vi "IIR Cascade Filter PtByPt.vi"(2 "initialize":bool, 3 "IIR Filter Cluster":T1, 5 "x":dbl format="%0.2f") -> (0 "error":i32, 1 "Filtered x":dbl format="%0.2f")   [LabVIEW 2020, in "NI_PtbyPt.lvlib"]
doc: "Filters <B>x</B> using the cascade form of the IIR filter specified by the <B>IIR Filter Cluster</B>."
uses:
  NI_PtbyPt.lvlib
  IIR Cascade Filter (DBL).vi
  NI_AALBase.lvlib
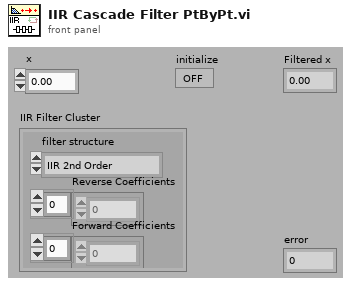
[diagram p1: front panel]
types:
  T1 = cluster{"filter structure":enum32{"IIR 2nd Order", "IIR 4th Order"}, "Reverse Coefficients":dbl[], "Forward Coefficients":dbl[]}
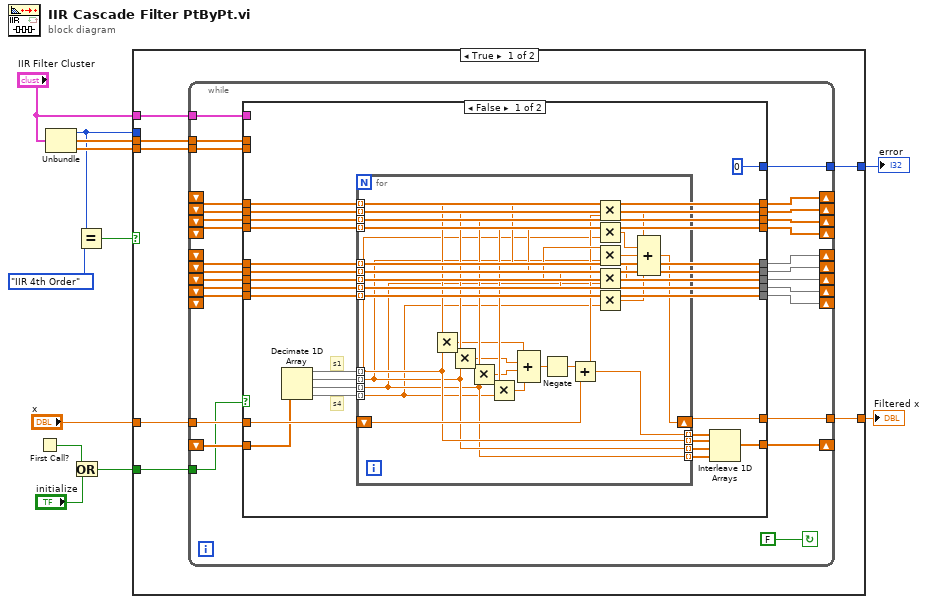
[diagram p0: block diagram]
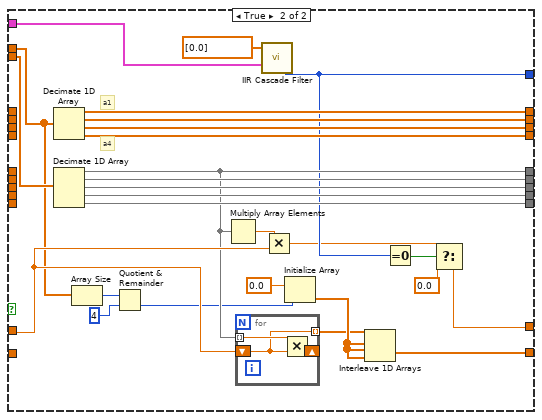
[diagram p2: hidden frame]
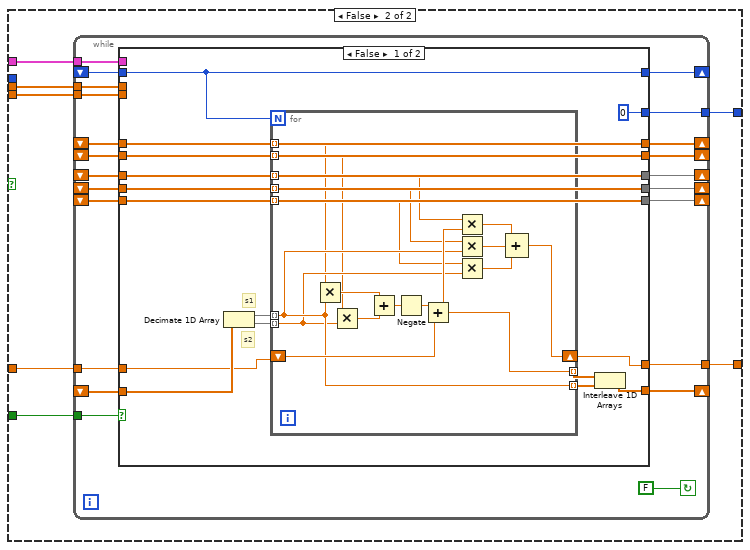
[diagram p3: hidden frame]
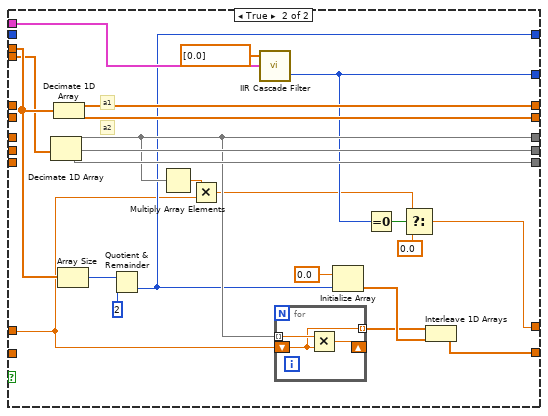
[diagram p4: hidden frame]
diagram:
  n1 = First Call?() -> (First Call?: T/F=w4:bool)
  n2 = Unbundle("IIR Filter Cluster") -> ("filter structure"=w9:enum32{"IIR 2nd Order", "IIR 4th Order"}, "Reverse Coefficients"=w10:dbl[], "Forward Coefficients"=w11:dbl[])
  n3 = Or(x=w4, y="initialize") -> (x .or. y?=w5:bool)
  n4 = Equal?(x=w9, y=enum32{"IIR 2nd Order", "IIR 4th Order"}."IIR 4th Order") -> (x = y?=w7:bool)
  n5 = case shown="True" w7 {
    tunnel: "x" -> [w18 w132]
    tunnel: w11 -> [w16 w130]
    tunnel: w9 -> [_ _]
    tunnel: w10 -> [w17 w131]
    tunnel: [w15 w129] -> w6
    tunnel: w5 -> [w19 w133]
    tunnel: "IIR Filter Cluster" -> [w14 w128]
    tunnel: [w13 w127] -> w2
    frame True {
      n6 = while {
        tunnel: [w21] -> w13
        tunnel: w14 -> [w22]
        tunnel: [w25] -> w15
        shift-left: _ -> [w26]
        shift-right: [w24] -> _
        shift-left: _ -> [w27]
        shift-right: [w28] -> _
        shift-left: _ -> [w29]
        shift-right: [w31] -> _
        shift-left: _ -> [w30]
        shift-right: [w32] -> _
        shift-left: _ -> [w33]
        shift-right: [w34] -> _
        tunnel: w18 -> [w35]
        tunnel: w17 -> [w36]
        shift-left: _ -> [w37]
        shift-right: [w39] -> _
        shift-left: _ -> [w38]
        shift-right: [w40] -> _
        shift-left: _ -> [w42]
        shift-right: [w45] -> _
        shift-left: _ -> [w41]
        shift-right: [w44] -> _
        shift-left: _ -> [w43]
        shift-right: [w46] -> _
        tunnel: w16 -> [w47]
        tunnel: w19 -> [w20]
        stop <- FALSE continue-if-true
        n7 = case shown="False" w20 {
          tunnel: w47 -> [_ w112]
          tunnel: [w64 w119] -> w46
          tunnel: [w63 w118] -> w45
          tunnel: [w62 w117] -> w44
          tunnel: w43 -> [w64 _]
          tunnel: w42 -> [w63 _]
          tunnel: w41 -> [w62 _]
          tunnel: [w67 w121] -> w40
          tunnel: [w66 w120] -> w39
          tunnel: w38 -> [w67 _]
          tunnel: w37 -> [w66 _]
          tunnel: w36 -> [_ w100]
          tunnel: w35 -> [w56 w110]
          tunnel: [w68 w122] -> w34
          tunnel: w33 -> [w68 _]
          tunnel: [w65 w109] -> w32
          tunnel: [w61 w116] -> w31
          tunnel: w30 -> [w65 _]
          tunnel: w29 -> [w61 _]
          tunnel: [w69 w123] -> w28
          tunnel: w27 -> [w69 _]
          tunnel: [w54 w102] -> w25
          tunnel: w26 -> [w55 _]
          tunnel: [w49 w111] -> w24
          tunnel: w22 -> [_ w107]
          tunnel: [0 ("error") w105] -> w21
          frame False {
            # "s4"
            # "s1"
            n8 = Decimate 1D Array(w55) -> (w60:dbl[], w59:dbl[], w58:dbl[], w57:dbl[])
            n9 = for {
              tunnel: w67 -> [w94] mode=indexing
              tunnel: w66 -> [w93] mode=indexing
              tunnel: w64 -> [w85] mode=indexing
              tunnel: w63 -> [w84] mode=indexing
              tunnel: w62 -> [w83] mode=indexing
              tunnel: w68 -> [w95] mode=indexing
              tunnel: w61 -> [w82] mode=indexing
              tunnel: w69 -> [w96] mode=indexing
              tunnel: w65 -> [w86] mode=indexing
              tunnel: w60 -> [w73] mode=indexing
              tunnel: w59 -> [w72] mode=indexing
              tunnel: w58 -> [w71] mode=indexing
              tunnel: w57 -> [w70] mode=indexing
              tunnel: [w74] -> w53 mode=indexing
              tunnel: [w71] -> w50 mode=indexing
              tunnel: [w72] -> w51 mode=indexing
              tunnel: [w73] -> w52 mode=indexing
              shift-right: [w75] -> w54
              shift-left: w56 -> [w76]
              n10 = Multiply(x=w96, y=w73) -> (x*y=w92:dbl)
              n11 = Multiply(x=w95, y=w72) -> (x*y=w91:dbl)
              n12 = Multiply(x=w94, y=w71) -> (x*y=w90:dbl)
              n13 = Multiply(x=w93, y=w70) -> (x*y=w89:dbl)
              n14 = Compound Arithmetic op=ADD(w92, w91, w90, w89) -> (w88:dbl)
              n15 = Negate(x=w88) -> (-x=w87:dbl)
              n16 = Add(x=w87, y=w76) -> (x+y=w74:dbl)
              n17 = Multiply(x=w86, y=w74) -> (x*y=w81:dbl)
              n18 = Multiply(x=w85, y=w73) -> (x*y=w80:dbl)
              n19 = Multiply(x=w84, y=w72) -> (x*y=w79:dbl)
              n20 = Multiply(x=w83, y=w71) -> (x*y=w78:dbl)
              n21 = Multiply(x=w82, y=w70) -> (x*y=w77:dbl)
              n22 = Compound Arithmetic op=ADD(w81, w80, w79, w78, w77) -> (w75:dbl)
            }
            n23 = Interleave 1D Arrays(w53, w52, w51, w50) -> (w49:dbl[])
          }
          frame True {
            # "a4"
            # "a1"
            n24 = Decimate 1D Array(w100) -> (w123:dbl[], w122:dbl[], w121:dbl[], w120:dbl[])
            n25 = Decimate 1D Array(w112) -> (w109:dbl[], w119:dbl[], w118:dbl[], w117:dbl[], w116:dbl[])
            n26 = Array Size(array=w100) -> (size(s)=w99:i32)
            n27 = Quotient & Remainder(x=w99, y=4) -> (floor(x/y)=w97:i32)  [unwired: 1 out]
            n28 = Multiply Array Elements(1:w109) -> (0:w115:dbl)
            n29 = for {
              shift-right: [w125] -> _
              shift-left: w110 -> [w124]
              tunnel: w109 -> [w126] mode=indexing
              tunnel: [w124] -> w108 mode=indexing
              n30 = Multiply(x=w126, y=w124) -> (x*y=w125:dbl)
            }
            n31 = call-poly "IIR Cascade Filter.vi"("IIR Filter Cluster"=w107, "X"=dbl[] [0.0]) -> ("error"=w105:i32)  [unwired: 1 in, 1 out]
            n32 = Multiply(x=w115, y=w110) -> (x*y=w103:dbl)
            n33 = Initialize Array(0.0 ("Element Data"), w97) -> (w113:dbl[])
            n34 = Interleave 1D Arrays(w108, w113, w113, w113) -> (w111:dbl[])
            n35 = Equal To 0?(x=w105) -> (x = 0?=w104:bool)
            n36 = Select(t=w103, s=w104, f=0.0) -> (s? t:f=w102:dbl)
          }
        }
      }
    }
    frame False {
      n37 = while {
        tunnel: [w135] -> w127
        tunnel: w128 -> [w136]
        tunnel: [w139] -> w129
        shift-left: _ -> [w140]
        shift-right: [w138] -> _
        shift-left: _ -> [w143]
        shift-right: [w144] -> _
        shift-left: _ -> [w145]
        shift-right: [w146] -> _
        shift-left: _ -> [w147]
        shift-right: [w148] -> _
        tunnel: w132 -> [w149]
        tunnel: w131 -> [w150]
        shift-left: _ -> [w151]
        shift-right: [w153] -> _
        shift-left: _ -> [w152]
        shift-right: [w154] -> _
        shift-left: _ -> [w141]
        shift-right: [w142] -> _
        tunnel: w130 -> [w155]
        tunnel: w133 -> [w134]
        stop <- FALSE continue-if-true
        n38 = case shown="False" w134 {
          tunnel: w155 -> [_ w194]
          tunnel: [w167 w208] -> w154
          tunnel: [w166 w207] -> w153
          tunnel: w152 -> [w167 _]
          tunnel: w151 -> [w166 _]
          tunnel: w150 -> [_ w202]
          tunnel: w149 -> [w157 w193]
          tunnel: [w164 w209] -> w148
          tunnel: w147 -> [w164 _]
          tunnel: [w168 w200] -> w146
          tunnel: w145 -> [w168 _]
          tunnel: [w165 w210] -> w144
          tunnel: w143 -> [w165 _]
          tunnel: [w169 w196] -> w142
          tunnel: w141 -> [w169 _]
          tunnel: [w158 w188] -> w139
          tunnel: w140 -> [w170 _]
          tunnel: [w159 w203] -> w138
          tunnel: w136 -> [_ w198]
          tunnel: [0 ("error") w192] -> w135
          frame False {
            # "s2"
            # "s1"
            n39 = Decimate 1D Array(w170) -> (w163:dbl[], w162:dbl[])
            n40 = for {
              N: w169 -> [_]
              tunnel: w163 -> [w177] mode=indexing
              tunnel: w162 -> [w176] mode=indexing
              tunnel: [w178] -> w161 mode=indexing
              tunnel: [w177] -> w160 mode=indexing
              shift-right: [w179] -> w158
              shift-left: w157 -> [w180]
              tunnel: w168 -> [w175] mode=indexing
              tunnel: w167 -> [w174] mode=indexing
              tunnel: w166 -> [w173] mode=indexing
              tunnel: w165 -> [w172] mode=indexing
              tunnel: w164 -> [w171] mode=indexing
              n41 = Multiply(x=w172, y=w177) -> (x*y=w187:dbl)
              n42 = Multiply(x=w171, y=w176) -> (x*y=w186:dbl)
              n43 = Add(x=w187, y=w186) -> (x+y=w185:dbl)
              n44 = Negate(x=w185) -> (-x=w184:dbl)
              n45 = Add(x=w184, y=w180) -> (x+y=w178:dbl)
              n46 = Multiply(x=w175, y=w178) -> (x*y=w183:dbl)
              n47 = Multiply(x=w174, y=w177) -> (x*y=w182:dbl)
              n48 = Multiply(x=w173, y=w176) -> (x*y=w181:dbl)
              n49 = Compound Arithmetic op=ADD(w183, w182, w181) -> (w179:dbl)
            }
            n50 = Interleave 1D Arrays(w161, w160) -> (w159:dbl[])
          }
          frame True {
            # "a2"
            # "a1"
            n51 = Decimate 1D Array(w194) -> (w200:dbl[], w208:dbl[], w207:dbl[])
            n52 = Decimate 1D Array(w202) -> (w210:dbl[], w209:dbl[])
            n53 = Array Size(array=w202) -> (size(s)=w195:i32)
            n54 = Quotient & Remainder(x=w195, y=2) -> (floor(x/y)=w196:i32)  [unwired: 1 out]
            n55 = Multiply Array Elements(1:w200) -> (0:w206:dbl)
            n56 = Multiply(x=w206, y=w193) -> (x*y=w190:dbl)
            n57 = call-poly "IIR Cascade Filter.vi"("IIR Filter Cluster"=w198, "X"=dbl[] [0.0]) -> ("error"=w192:i32)  [unwired: 1 in, 1 out]
            n58 = for {
              shift-right: [w212] -> _
              shift-left: w193 -> [w211]
              tunnel: w200 -> [w213] mode=indexing
              tunnel: [w211] -> w199 mode=indexing
              n59 = Multiply(x=w213, y=w211) -> (x*y=w212:dbl)
            }
            n60 = Initialize Array(0.0 ("Element Data"), w196) -> (w201:dbl[])
            n61 = Equal To 0?(x=w192) -> (x = 0?=w191:bool)
            n62 = Select(t=w190, s=w191, f=0.0) -> (s? t:f=w188:dbl)
            n63 = Interleave 1D Arrays(w199, w201) -> (w203:dbl[])
          }
        }
      }
    }
  }
  "Filtered x" <- w6
  "error" <- w2
